vi "retrieve token.vi"(8 "error in (no error)":errorcluster, 10 "Token Request URI":string, 11 "Oauth2 in":refnum<class "Oauth2.lvclass">) -> (0 "error out":errorcluster, 1 "Response":string, 2 "Header":string, 3 "Oauth2 out":refnum<class "Oauth2.lvclass">)   [LabVIEW 2020, in "Oauth2.lvclass"]
uses:
  Oauth2.lvclass
  Oauth2.lvclass/Oauth2.ctl
  OauthClient/OAuthClient.lvclass
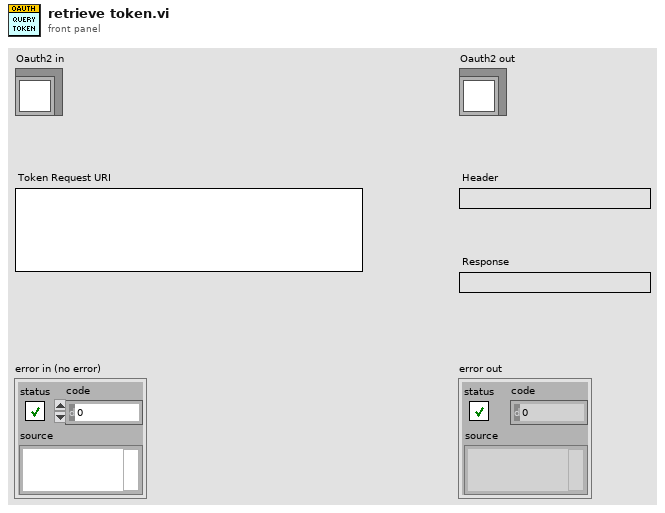
[diagram p1: front panel]
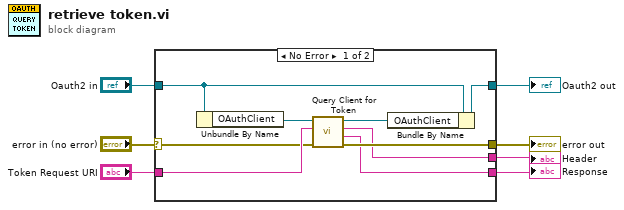
[diagram p0: block diagram]
diagram:
  n1 = case shown="No Error" "error in (no error)" {
    selector: "error in (no error)" -> [w11 w18]
    tunnel: [w10 w18] -> w6
    tunnel: [w15 w17] -> w4
    tunnel: "Oauth2 in" -> [w16 w17]
    tunnel: [w9 _] -> w3
    tunnel: "Token Request URI" -> [w12 _]
    tunnel: [w8 _] -> w1
    frame No Error {
      n2 = Unbundle By Name(w16) -> ("OAuthClient"=w14:refnum<class "OAuthClient.lvclass">)
      n3 = call-dynamic "Query Client for Token.vi"("error in (no error)"=w11, "Request URI"=w12, "OAuthClient in"=w14) -> ("error out"=w10:errorcluster, "Body"=w9:string, "Header"=w8:string, "OAuthClient out"=w13:refnum<class "OAuthClient.lvclass">)  [unwired: 5 in]
      n4 = Bundle By Name(cluster=w16, "OAuthClient"=w13) -> (w15:refnum<class "Oauth2.lvclass">)
    }
    frame Error {
    }
  }
  "error out" <- w6
  "Oauth2 out" <- w4
  "Response" <- w3
  "Header" <- w1
